vi "Grabber Position to Angles.vi"(8 "Forearm Length":dbl, 9 "Backarm Length":dbl, 10 "Y Initial":dbl, 11 "X Initial":dbl) -> (0 "Forearm Angle\nDegrees 2":dbl format="%.2f", 1 "Backarm Angle\nDegrees 2":dbl format="%.2f", 2 "Forearm Angle\nDegrees 1":dbl format="%.2f", 3 "Backarm Angle\nDegrees 1":dbl format="%.2f")   [LabVIEW 2017]
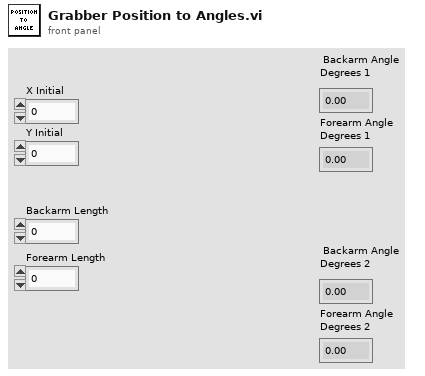
[diagram p1: front panel]
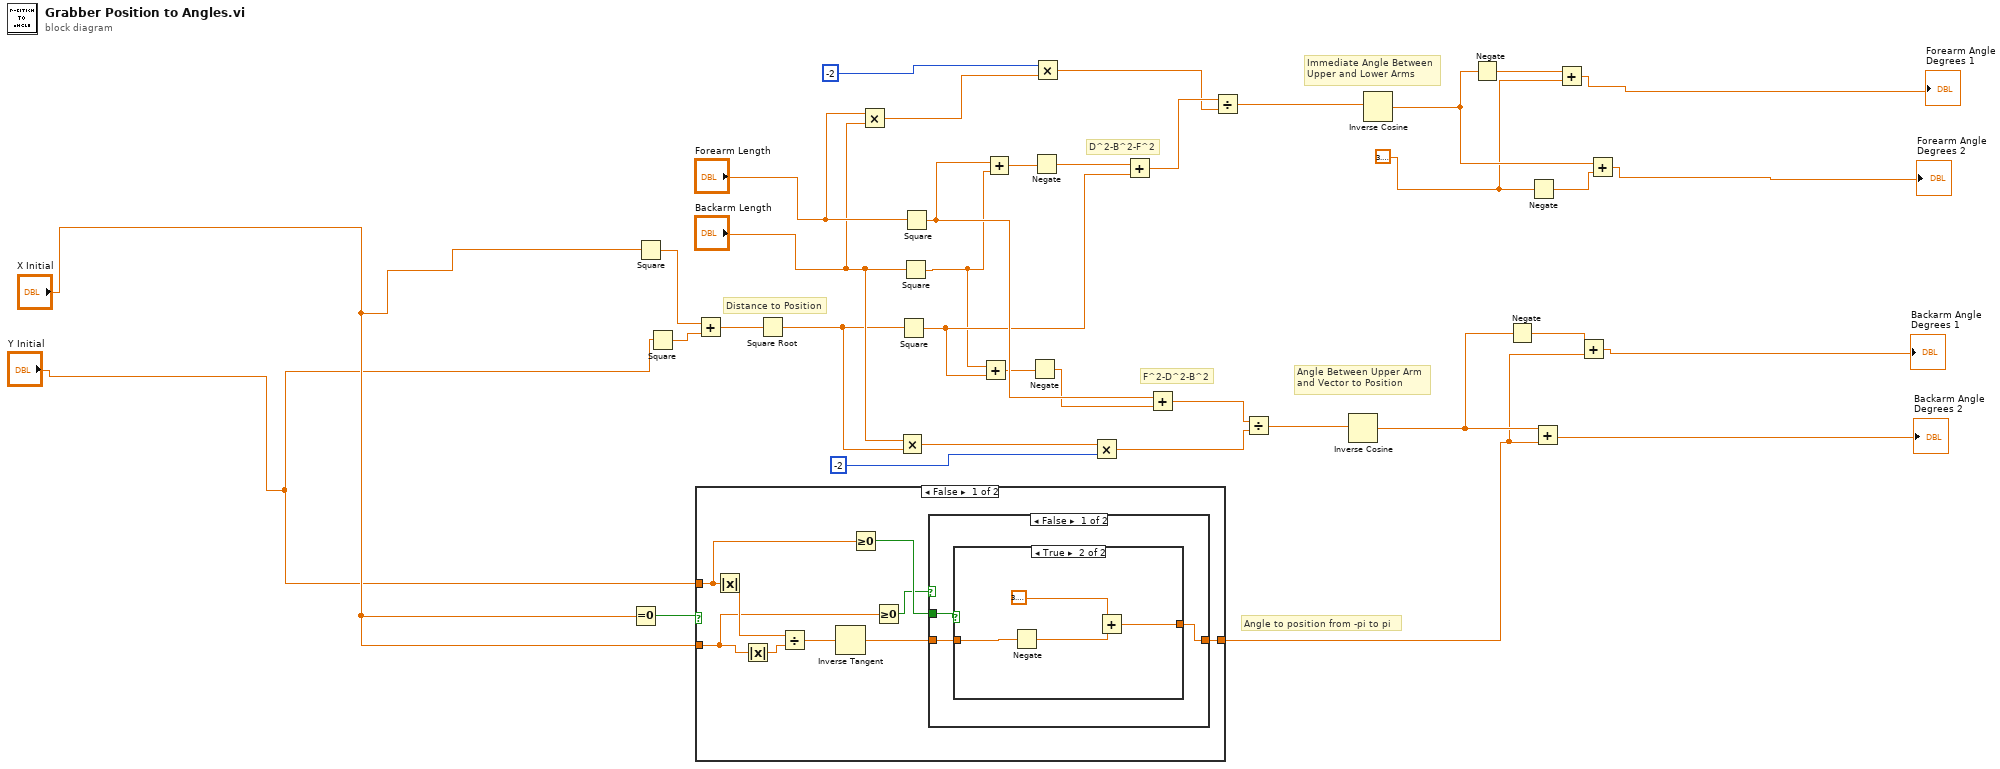
[diagram p0: block diagram]
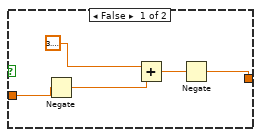
[diagram p2: hidden frame]
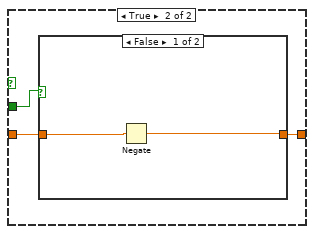
[diagram p3: hidden frame]
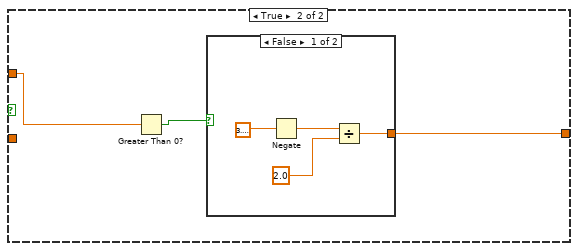
[diagram p5: hidden frame]
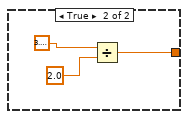
[diagram p6: hidden frame]
diagram:
  w12 = 3.141592653589793
  # "Angle Between Upper Arm\nand Vector to Position"
  # "Immediate Angle Between\nUpper and Lower Arms"
  # "F^2-D^2-B^2"
  # "D^2-B^2-F^2"
  # "Distance to Position"
  # "Angle to position from -pi to pi"
  n1 = Equal To 0?(x="X Initial") -> (x = 0?=w7:bool)
  n2 = Square(x="X Initial") -> (x^2=w37:dbl)
  n3 = Square(x="Y Initial") -> (x^2=w36:dbl)
  n4 = case shown="False" w7 {
    tunnel: "Y Initial" -> [w42 w66]
    tunnel: [w40 w65] -> w8
    tunnel: "X Initial" -> [w41 _]
    frame False {
      n5 = Absolute Value(x=w42) -> (abs(x)=w43:dbl)
      n6 = Absolute Value(x=w41) -> (abs(x)=w44:dbl)
      n7 = Divide(x=w43, y=w44) -> (x/y=w45:dbl)
      n8 = Inverse Tangent(1:w45) -> (0:w46:dbl)
      n9 = Greater Or Equal To 0?(x=w42) -> (x >= 0?=w39:bool)
      n10 = Greater Or Equal To 0?(x=w41) -> (x >= 0?=w38:bool)
      n11 = case shown="False" w38 {
        tunnel: w39 -> [w49 w61]
        tunnel: w46 -> [w48 w60]
        tunnel: [w47 w59] -> w40
        frame False {
          n12 = case shown="True" w49 {
            tunnel: w48 -> [w52 w58]
            tunnel: [w50 w55] -> w47
            frame False {
              n13 = Negate(x=w52) -> (-x=w54:dbl)
              n14 = Add(x=3.141592653589793, y=w54) -> (x+y=w51:dbl)
              n15 = Negate(x=w51) -> (-x=w50:dbl)
            }
            frame True {
              n16 = Negate(x=w58) -> (-x=w56:dbl)
              n17 = Add(x=3.141592653589793, y=w56) -> (x+y=w55:dbl)
            }
          }
        }
        frame True {
          n18 = case shown="False" w61 {
            tunnel: w60 -> [w63 w64]
            tunnel: [w62 w64] -> w59
            frame False {
              n19 = Negate(x=w63) -> (-x=w62:dbl)
            }
            frame True {
            }
          }
        }
      }
    }
    frame True {
      n20 = Greater Than 0?(x=w66) -> (x > 0?=w67:bool)
      n21 = case shown="False" w67 {
        tunnel: [w69 w74] -> w65
        frame False {
          n22 = Negate(x=3.141592653589793) -> (-x=w70:dbl)
          n23 = Divide(x=w70, y=2.0) -> (x/y=w69:dbl)
        }
        frame True {
          n24 = Divide(x=3.141592653589793, y=2.0) -> (x/y=w74:dbl)
        }
      }
    }
  }
  n25 = Add(x=w37, y=w36) -> (x+y=w35:dbl)
  n26 = Square Root(x=w35) -> (sqrt(x)=w32:dbl)
  n27 = Multiply(x="Forearm Length", y="Backarm Length") -> (x*y=w31:dbl)
  n28 = Multiply(x="Backarm Length", y=w32) -> (x*y=w28:dbl)
  n29 = Square(x=w32) -> (x^2=w24:dbl)
  n30 = Square(x="Backarm Length") -> (x^2=w23:dbl)
  n31 = Square(x="Forearm Length") -> (x^2=w25:dbl)
  n32 = Add(x=w23, y=w24) -> (x+y=w21:dbl)
  n33 = Add(x=w25, y=w23) -> (x+y=w27:dbl)
  n34 = Negate(x=w21) -> (-x=w22:dbl)
  n35 = Negate(x=w27) -> (-x=w26:dbl)
  n36 = Multiply(x=-2, y=w31) -> (x*y=w19:dbl)
  n37 = Multiply(x=w28, y=-2) -> (x*y=w17:dbl)
  n38 = Add(x=w26, y=w24) -> (x+y=w20:dbl)
  n39 = Add(x=w25, y=w22) -> (x+y=w18:dbl)
  n40 = Divide(x=w20, y=w19) -> (x/y=w16:dbl)
  n41 = Divide(x=w18, y=w17) -> (x/y=w15:dbl)
  n42 = Inverse Cosine(1:w15) -> (0:w10:dbl)
  n43 = Inverse Cosine(1:w16) -> (0:w14:dbl)
  n44 = Negate(x=w14) -> (-x=w13:dbl)
  n45 = Negate(x=w10) -> (-x=w9:dbl)
  n46 = Negate(x=w12) -> (-x=w11:dbl)
  n47 = Add(x=w10, y=w8) -> (x+y=→"Backarm Angle\nDegrees 2":dbl)
  n48 = Add(x=w13, y=w12) -> (x+y=→"Forearm Angle\nDegrees 1":dbl)
  n49 = Add(x=w9, y=w8) -> (x+y=→"Backarm Angle\nDegrees 1":dbl)
  n50 = Add(x=w14, y=w11) -> (x+y=→"Forearm Angle\nDegrees 2":dbl)
